vi "Disabled Value.vi"(4 "Disabled":bool, 5 "Grayed Out (T)":bool=TRUE) -> (7 "Disabled Value":T1(ring))   [LabVIEW 2020, in "VolatusGUI.lvlib" / "GUI Element.lvclass"]
uses:
  GUI Element.lvclass
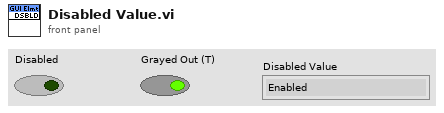
[diagram p1: front panel]
types:
  T1 = enum8{"Enabled", "Disabled", "Disabled and Grayed Out"}
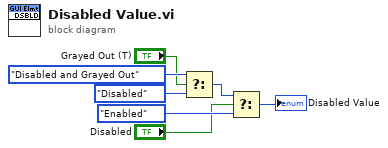
[diagram p0: block diagram]
diagram:
  n1 = Select(t=T1."Disabled and Grayed Out", s="Grayed Out (T)", f=T1."Disabled" ("t")) -> (s? t:f=w3:T1)
  n2 = Select(t=w3, s="Disabled", f=T1."Enabled" ("Disabled")) -> (s? t:f=→"Disabled Value":T1)
